vi "CreateTextFile.vi"(11 "Input File Path":path) -> ()   [LabVIEW 2019, in "FileUtilities.lvlib"]
uses:
  FileUtilities.lvlib
  GraphUtilities/GraphUtilities.lvclass
panel:
  in  "GraphUtilities.lvclass 2":refnum<class "GraphUtilities.lvclass">
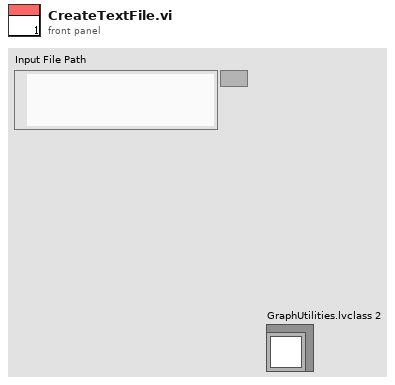
[diagram p1: front panel]
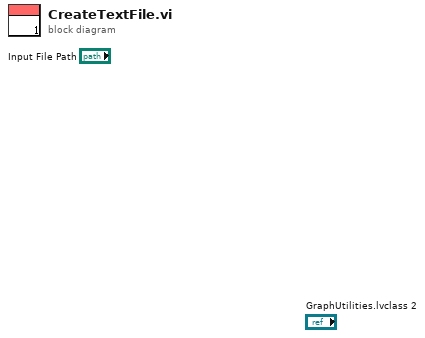
[diagram p0: block diagram]
diagram:
